vi "Configured Connection.vi"(8 "error in (no error)":errorcluster, 11 "TCPConfigPanel in":refnum<class "TCPConfigPanel.lvclass">) -> (0 "error out":errorcluster, 2 "Configured Connection":refnum<class "Connection.lvclass">, 3 "TCPConfigPanel out":refnum<class "TCPConfigPanel.lvclass">)   [LabVIEW 2020, in "LV-Term.lvlib" / "TCPConfigPanel.lvclass"]
uses:
  TCPConfigPanel.lvclass
  <vilib>/IlluminatedG/lv-stream-tcp/TCP Client/TCP Client.lvclass
  C:/Program Files (x86)/National Instruments/LabVIEW 2020/vi.lib/IlluminatedG/lv-stream/Endpoint/Endpoint.lvclass
  TCPConfigPanel.lvclass/TCPConfigPanel.ctl
  <vilib>/IlluminatedG/lv-stream-tcp/Stream-TCP.lvlib
  <vilib>/IlluminatedG/lv-stream/Endpoint/Endpoint.lvclass
  C:/Program Files (x86)/National Instruments/LabVIEW 2020/vi.lib/IlluminatedG/lv-stream/Connection/Connection.lvclass
  C:/Program Files (x86)/National Instruments/LabVIEW 2020/vi.lib/IlluminatedG/lv-stream-tcp/TCP Client/TCP Client.lvclass
  <vilib>/IlluminatedG/lv-stream/Connection/Connection.lvclass
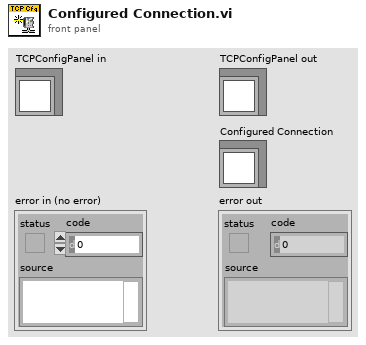
[diagram p1: front panel]
types:
  T1 = typedef "LV-Term.lvlib/TCPConfigPanel.lvclass/Ref Data.ctl" = cluster{"Host":string, "Port":u16}
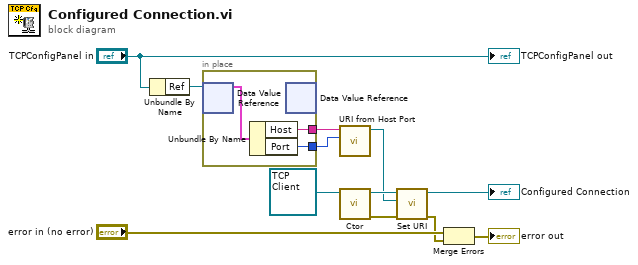
[diagram p0: block diagram]
diagram:
  n1 = Unbundle By Name("TCPConfigPanel in") -> ("Ref"=w11:refnum<data-value>)
  n2 = in-place {
    in-place-border: [w14] -> w9
    in-place-border: [w13] -> w8
    n3 = in-place-dvr #1(w11) -> (w15:T1)  [unwired: 1 out]
    n4 = Unbundle By Name(w15) -> ("Host"=w14:string, "Port"=w13:u16)
    n5 = in-place-dvr #1() -> ()  [unwired: 1 in, 2 out]
  }
  n6 = call <vilib>:"URI from Host Port.vi"("Port"=w8, "Host"=w9) -> ("URI"=w5:refnum<class "URI.lvclass">)  [unwired: 9 in]
  n7 = call-dynamic "Ctor.vi"("TCP Client in"=refnum<class "TCP Client.lvclass"> refnum) -> ("error out"=w4:errorcluster, "TCP Client out"=w7:refnum<class "TCP Client.lvclass">)  [unwired: 9 in]
  n8 = call <vilib>:"Set URI.vi"("error in (no error)"=w4, "URI"=w5, "Endpoint in"=w7) -> ("error out"=w2:errorcluster, "Endpoint out"=→"Configured Connection":refnum<class "TCP Client.lvclass">)  [unwired: 7 in]
  n9 = Merge Errors("error in (no error)", w2) -> (→"error out":errorcluster)
  "TCPConfigPanel out" <- "TCPConfigPanel in"
